vi "VI Tree.vi"   [LabVIEW 2016, in "Andeen-Hagerling 2550.lvlib"]
doc: "This is the instrument driver for the <INSTRUMENT NAME>. The VI Tree displays all the user-callable VIs of the instrument driver in an organized table."
uses:
  Andeen-Hagerling 2550.lvlib
panel:
  # "(c) 2007 Andeen-Hagerling, Inc.  ALL RIGHTS RESERVED."
  # "SEE DIAGRAM\nFOR VI TREE."
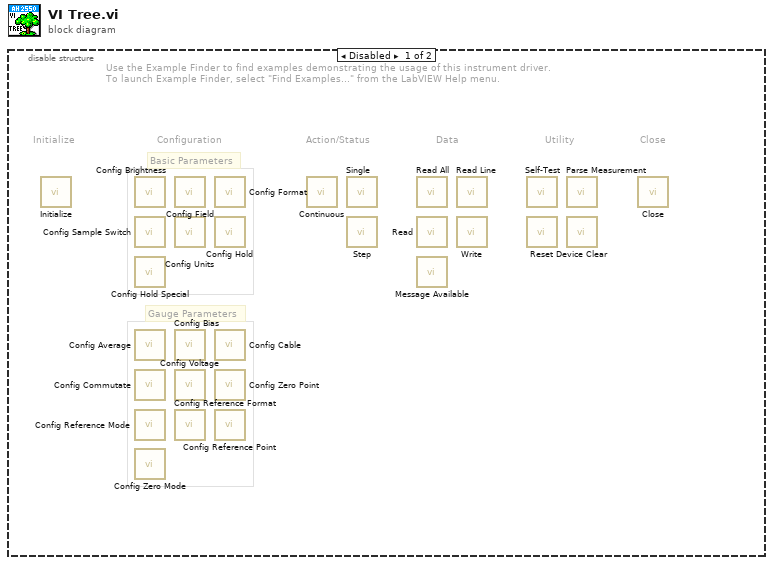
[diagram p0: block diagram]
diagram:
  n1 = disable-structure shown="Disabled" {
    frame Disabled {
      # "Gauge Parameters"
      # "Basic Parameters"
      # "Use the Example Finder to find examples demonstrating the usage of this instrument driver.\nTo launch Example Finder, select \"Find Examples...\" from the LabVIEW Help menu."
      # "Configuration"
      # "Utility"
      # "Data"
      # "Action/Status"
      # "Close"
      # "Initialize"
      n2 = call "Initialize.vi"() -> ()  [unwired: 10 in, 2 out]
      n3 = call "Config Brightness.vi"() -> ()  [unwired: 10 in, 2 out]
      n4 = call "Config Sample Switch.vi"() -> ()  [unwired: 10 in, 2 out]
      n5 = call "Config Hold Special.vi"() -> ()  [unwired: 10 in, 2 out]
      n6 = call "Config Average.vi"() -> ()  [unwired: 10 in, 2 out]
      n7 = call "Config Commutate.vi"() -> ()  [unwired: 10 in, 2 out]
      n8 = call "Config Reference Mode.vi"() -> ()  [unwired: 10 in, 2 out]
      n9 = call "Config Zero Mode.vi"() -> ()  [unwired: 10 in, 2 out]
      n10 = call "Config Field.vi"() -> ()  [unwired: 10 in, 2 out]
      n11 = call "Config Units.vi"() -> ()  [unwired: 10 in, 2 out]
      n12 = call "Config Bias.vi"() -> ()  [unwired: 10 in, 2 out]
      n13 = call "Config Voltage.vi"() -> ()  [unwired: 10 in, 2 out]
      n14 = call "Config Reference Format.vi"() -> ()  [unwired: 10 in, 2 out]
      n15 = call "Config Format.vi"() -> ()  [unwired: 10 in, 2 out]
      n16 = call "Config Hold.vi"() -> ()  [unwired: 10 in, 2 out]
      n17 = call "Config Cable.vi"() -> ()  [unwired: 10 in, 2 out]
      n18 = call "Config Zero Point.vi"() -> ()  [unwired: 10 in, 2 out]
      n19 = call "Config Reference Point.vi"() -> ()  [unwired: 10 in, 2 out]
      n20 = call "Continuous.vi"() -> ()  [unwired: 10 in, 2 out]
      n21 = call "Single.vi"() -> ()  [unwired: 10 in, 2 out]
      n22 = call "Step.vi"() -> ()  [unwired: 10 in, 2 out]
      n23 = call "Read All.vi"() -> ()  [unwired: 8 in, 4 out]
      n24 = call "Read.vi"() -> ()  [unwired: 8 in, 4 out]
      n25 = call "Message Available.vi"() -> ()  [unwired: 9 in, 3 out]
      n26 = call "Read Line.vi"() -> ()  [unwired: 7 in, 5 out]
      n27 = call "Write.vi"() -> ()  [unwired: 10 in, 2 out]
      n28 = call "Self-Test.vi"() -> ()  [unwired: 8 in, 4 out]
      n29 = call "Reset.vi"() -> ()  [unwired: 10 in, 2 out]
      n30 = call "Parse Measurement.vi"() -> ()  [unwired: 11 in, 9 out]
      n31 = call "Device Clear.vi"() -> ()  [unwired: 10 in, 2 out]
      n32 = call "Close.vi"() -> ()  [unwired: 11 in, 1 out]
    }
    frame Enabled {
    }
  }
